vi "Examples.vi"() -> ()   [LabVIEW 2020, in "Examples.lvlib"]
uses:
  classes/Dual/Dual.lvclass/Dual.ctl
  classes/Dual/Add infinitesimal to Double.vi
  classes/Dual/Read Dual Part.vi
  classes/Dual/Dual to Double.vi
  Automatic Differentiation/Evaluate Function.vi/9b1629ae-3de0-49eb-9b0a-cc9e581fb6c0.vi
  Automatic Differentiation/Evaluate Function.vi/9b1629ae-3de0-49eb-9b0a-cc9e581fb6c0.vi/5957e011-cf56-4527-b6ed-13c3a4ca997b.vi
  classes/Dual/Write a.vi
  classes/Dual/Dual.lvclass
  Examples.lvlib
  Automatic Differentiation/Automatic Differentiation.lvlib
  Tests/Tests.lvlib
panel:
  in  "Initial guess":dbl=5.0 format="%#_13g"
  in  "Iterations [n]":i32=2
  out "x_n":dbl
  out "f(x) 3":dbl
  out "f'(x) 3":dbl
  out "f(x) 2":dbl
  out "f'(x) 2":dbl
  out "f'(x)":dbl
  out "f(x)":dbl
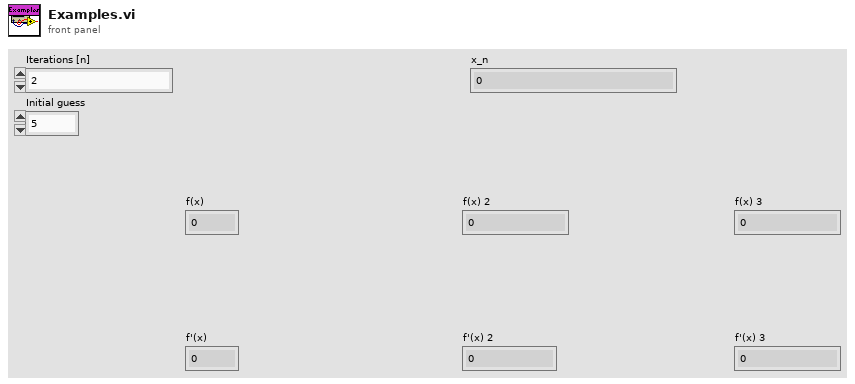
[diagram p1: front panel]
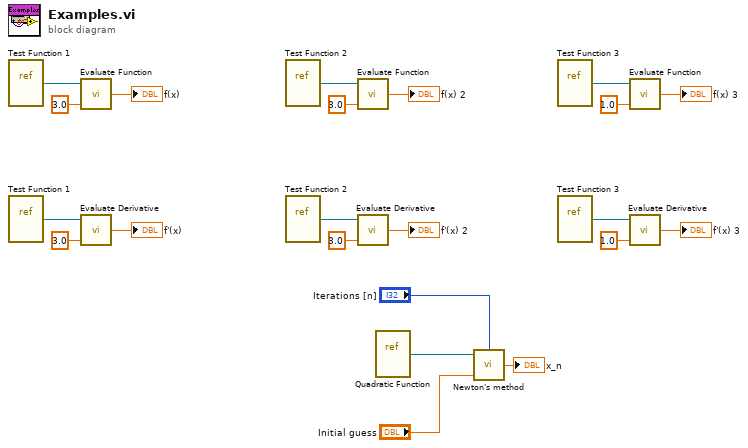
[diagram p0: block diagram]
diagram:
  n1 = vi-ref "Test Function 1.vi"() -> (w20:refnum<vi>)
  n2 = vi-ref "Test Function 1.vi"() -> (w19:refnum<vi>)
  n3 = call "Evaluate Function.vi"("x"=3.0, "Function Reference"=w20) -> ("f(x)"=→"f(x)":dbl)  [unwired: 1 in]
  n4 = call "Evaluate Derivative.vi"("x"=3.0, "Function Reference"=w19) -> ("f'(x)"=→"f'(x)":dbl)  [unwired: 1 in]
  n5 = vi-ref "Test Function 2.vi"() -> (w13:refnum<vi>)
  n6 = vi-ref "Test Function 2.vi"() -> (w14:refnum<vi>)
  n7 = call "Evaluate Function.vi"("x"=3.0, "Function Reference"=w13) -> ("f(x)"=→"f(x) 2":dbl)  [unwired: 1 in]
  n8 = call "Evaluate Derivative.vi"("x"=3.0, "Function Reference"=w14) -> ("f'(x)"=→"f'(x) 2":dbl)  [unwired: 1 in]
  n9 = vi-ref "Quadratic Function.vi"() -> (w4:refnum<vi>)
  n10 = call "Newton's method.vi"("Max Iterations (1,000)"="Iterations [n]", "Initial Guess"="Initial guess", "Function Reference"=w4) -> ("x_n"=→"x_n":dbl)  [unwired: 1 in]
  n11 = vi-ref "Test Function 3.vi"() -> (w8:refnum<vi>)
  n12 = vi-ref "Test Function 3.vi"() -> (w7:refnum<vi>)
  n13 = call "Evaluate Function.vi"("x"=1.0, "Function Reference"=w8) -> ("f(x)"=→"f(x) 3":dbl)  [unwired: 1 in]
  n14 = call "Evaluate Derivative.vi"("x"=1.0, "Function Reference"=w7) -> ("f'(x)"=→"f'(x) 3":dbl)  [unwired: 1 in]
